vi "p11y2.vi"() -> ()   [LabVIEW 2020]
uses:
  P11Y2MRWORLDWIDE.vi
panel:
  out "GlobaalneArv":dbl
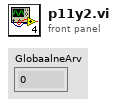
[diagram p1: front panel]
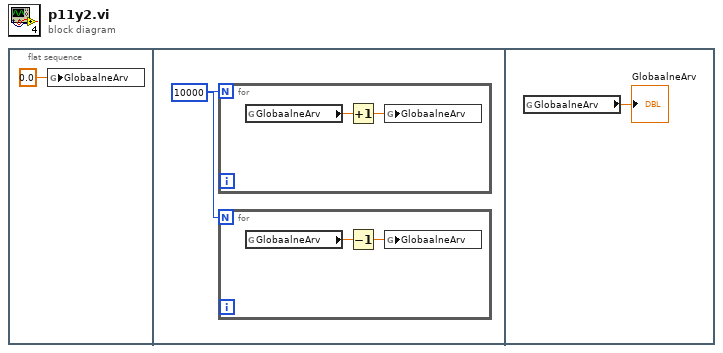
[diagram p0: block diagram]
diagram:
  n1 = flat-sequence {
    frame #0 {
      n2 = global write "P11Y2MRWORLDWIDE.vi" "GlobaalneArv"(0.0) -> ()
    }
    frame #1 {
      w2 = 10000
      n3 = for {
        N: w2 -> [_]
        n4 = global read "P11Y2MRWORLDWIDE.vi" "GlobaalneArv"() -> (w6:dbl)
        n5 = Increment(x=w6) -> (x+1=w5:dbl)
        n6 = global write "P11Y2MRWORLDWIDE.vi" "GlobaalneArv"(w5) -> ()
      }
      n7 = for {
        N: w2 -> [_]
        n8 = global read "P11Y2MRWORLDWIDE.vi" "GlobaalneArv"() -> (w4:dbl)
        n9 = Decrement(x=w4) -> (x-1=w3:dbl)
        n10 = global write "P11Y2MRWORLDWIDE.vi" "GlobaalneArv"(w3) -> ()
      }
    }
    frame #2 {
      n11 = global read "P11Y2MRWORLDWIDE.vi" "GlobaalneArv"() -> (→"GlobaalneArv":dbl)
    }
  }
